vi "AutoLoadRoutines.vi"(1 "Reload Routines":bool, 2 "Auto Routines Storage Directory":path=path "/home/lvuser/AutoRoutines") -> (0 "Auto Routines":T1)   [LabVIEW 2017]
uses:
  TypeDef/AutoRoutines.ctl
  TypeDef/AutoRoutineSet.ctl
  TypeDef/AutoStep.ctl
  TypeDef/AutoWaypointType.ctl
  Pathfinder/Pathfinder-LabVIEW/Pathfinder-Lib/VIs/Waypoint.ctl
  Implements/Arm/TypeDefs/ArmTargetPosition.ctl
  Implements/TypeDefs/IntakeState.ctl
  TypeDef/AutoStartingPositions.ctl
  e61514f7-18c3-42f3-b2a8-fda8a5312ef7.vi
  55916f22-7f41-4e59-abc4-9fcd15d20e92.vi
  058e71e0-aaa7-4a66-86c1-b77b5f723853.vi
  <vilib>/Utility/file.llb/Read Delimited Spreadsheet (DBL).vi
  Pathfinder/Pathfinder-LabVIEW/Pathfinder-Lib/Pathfinder.lvlib
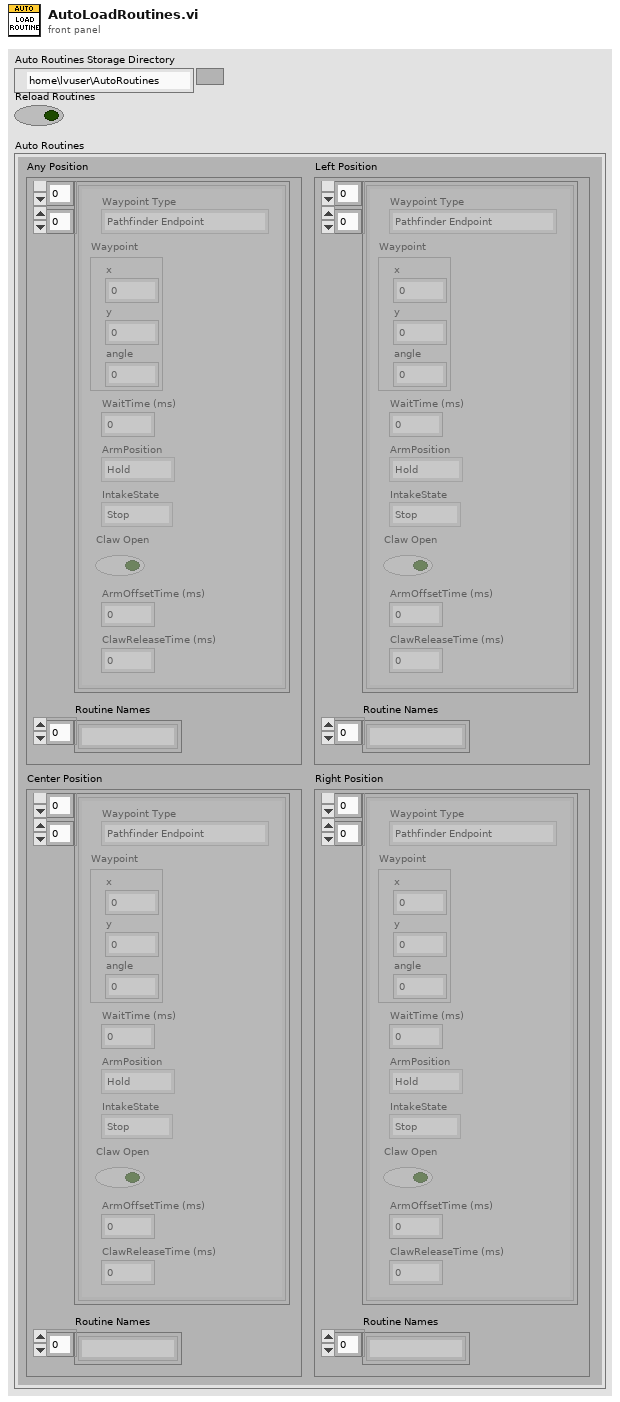
[diagram p1: front panel]
types:
  T1 = typedef "AutoRoutines.ctl" = cluster{"Any Position":T2, "Left Position":T2, "Center Position":T2, "Right Position":T2}
  T2 = typedef "AutoRoutineSet.ctl" = cluster{"Routines":T3[][], "Routine Names":string[]}
  T3 = typedef "AutoStep.ctl" = cluster{"Waypoint Type":T4, "Waypoint":T5, "WaitTime (ms)":u16, "ArmPosition":T6, "IntakeState":T7, "Claw Open":bool, "ArmOffsetTime (ms)":u16, "ClawReleaseTime (ms)":u16}
  T4 = typedef "AutoWaypointType.ctl" = enum16{"Pathfinder Endpoint", "Pathfinder Waypoint", "Zero-Radius Turn Endpoint", "Stationary", "Vision Assist Endpoint", "Stop"}
  T5 = typedef "Pathfinder.lvlib/Waypoint.ctl" = cluster{"x":dbl, "y":dbl, "angle":dbl}
  T6 = typedef "ArmTargetPosition.ctl" = enum16{"Hold", "Switch", "Scale Low", "Scale High", "Climb", "Back Place"}
  T7 = typedef "IntakeState.ctl" = enum16{"Stop", "Forward", "Reverse", "Forward Open"}
  T8 = typedef "AutoStartingPositions.ctl" = enum16{"Any", "Left", "Center", "Right"}
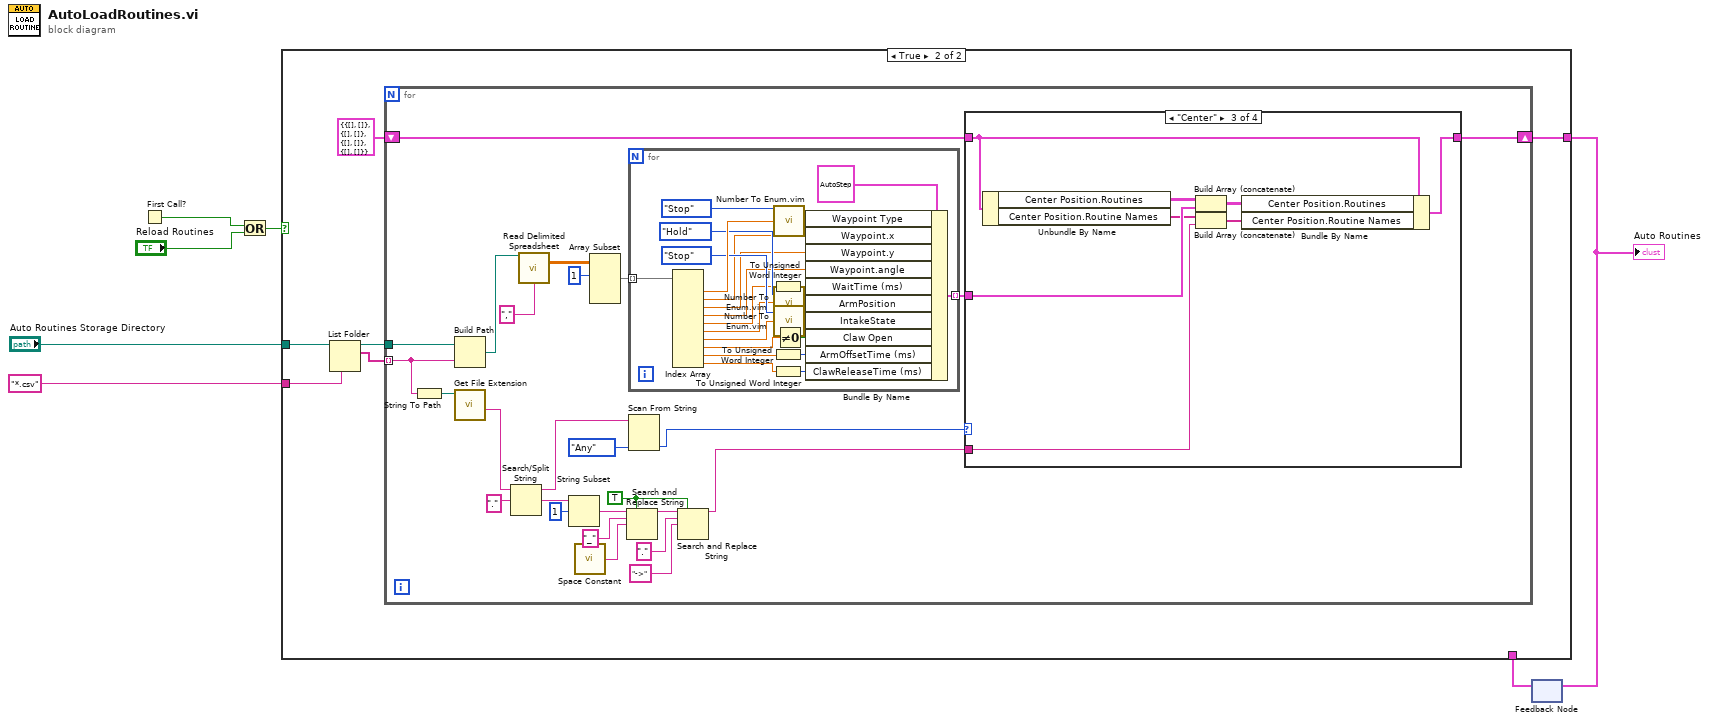
[diagram p0: block diagram]
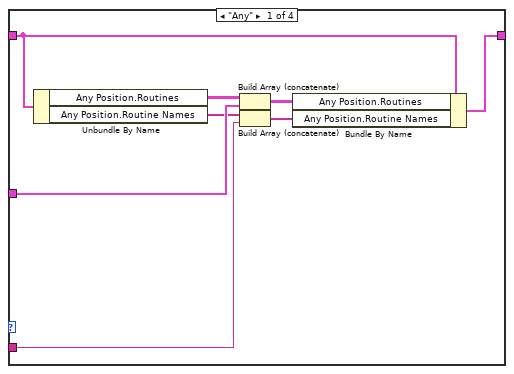
[diagram p3: hidden frame]
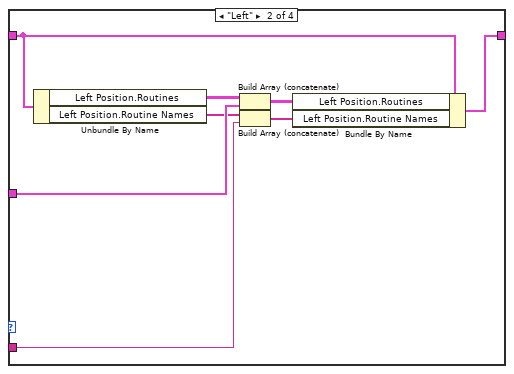
[diagram p4: hidden frame]
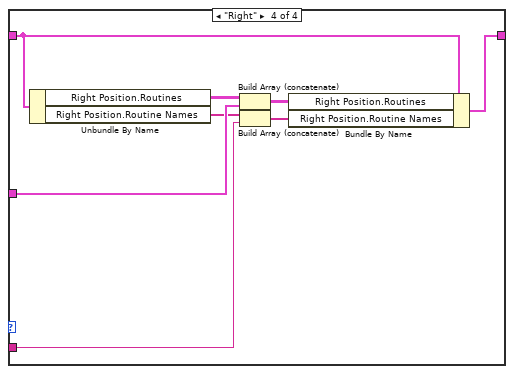
[diagram p5: hidden frame]
diagram:
  n1 = First Call?() -> (First Call?: T/F=w3:bool)
  n2 = Or(x=w3, y="Reload Routines") -> (x .or. y?=w5:bool)
  n3 = feedback #1() -> (w2:T1)  [unwired: 1 in]
  n4 = case shown="True" w5 {
    tunnel: "Auto Routines Storage Directory" -> [_ w14]
    tunnel: "*.csv" ("pattern") -> [_ w13]
    tunnel: [w8 w9] -> w1
    tunnel: w2 -> [w8 _]
    frame False {
    }
    frame True {
      n5 = List Folder(path=w14, pattern=w13) -> (path out=w12:path, filenames=w11:string[])  [unwired: 2 in, 2 out]
      n6 = for {
        tunnel: w12 -> [w37]
        tunnel: w11 -> [w15] mode=indexing
        shift-right: [w17] -> w9
        shift-left: T1 {"Any Position"={"Routines"=[], "Routine Names"=[]}, "Left Position"={"Routines"=[], "Routine Names"=[]}, "Center Position"={"Routines"=[], "Routine Names"=[]}, "Right Position"={"Routines"=[], "Routine Names"=[]}} ("Auto Routine") -> [w19]
        w27 = TRUE ("replace all? (F)")
        n7 = String To Path(string=w15) -> (path=w16:path)
        n8 = Build Path(base path=w37, name or relative path=w15) -> (appended path=w39:path)
        n9 = call <vilib>:"Get File Extension.vi"("file"=w16) -> ("filename without extension"=w36:string)  [unwired: 6 in, 4 out]
        n10 = Search/Split String(string=w36, search string/char (-)=".") -> (substring before match=w22:string, match + rest of string=w35:string)  [unwired: 1 in, 1 out]
        n11 = call-poly <vilib>:"Read Delimited Spreadsheet.vi"("file path (dialog if empty)"=w39, "delimiter (\\t)"="," ("delimiter (\\t)")) -> ("all rows"=w26:dbl[][])  [unwired: 8 in, 5 out]
        n12 = String Subset(string=w35, offset (0)=1) -> (substring=w33:string)  [unwired: 1 in]
        n13 = call <vilib>:"Space Constant.vi"() -> ("String"=w31:string)
        n14 = Array Subset(array=w26, index (row)=1 ("index")) -> (w24:dbl[][])  [unwired: 3 in]
        n15 = Search and Replace String(replace all?=w27, input string=w33, search string="_", replace string=w31) -> (result string=w30:string)  [unwired: 4 in, 3 out]
        n16 = for {
          tunnel: w24 -> [w95] mode=indexing
          tunnel: [w77] -> w18 mode=indexing
          n17 = Index Array(array=w95) -> (element #1=w90:dbl, element #2=w80:dbl, element #3=w79:dbl, element #4=w78:dbl, element #5=w82:dbl, element #6=w84:dbl, element #7=w85:dbl, element #8=w89:dbl, element #9=w76:dbl, element #10=w73:dbl)  [unwired: 10 in]
          n18 = To Unsigned Word Integer(number=w82) -> (unsigned 16bit integer=w81:u16)
          n19 = To Unsigned Word Integer(number=w76) -> (unsigned 16bit integer=w75:u16)
          n20 = To Unsigned Word Integer(number=w73) -> (unsigned 16bit integer=w74:u16)
          n21 = call "Number To Enum.vim"("number"=w90, "enum type"=AutoWaypointType."Stop" ("Waypoint Type")) -> ("number as enum"=w92:T4)
          n22 = call "Number To Enum.vim"("number"=w84, "enum type"=ArmTargetPosition."Hold" ("ArmPosition")) -> ("number as enum"=w86:T6)
          n23 = call "Number To Enum.vim"("number"=w85, "enum type"=IntakeState."Stop" ("IntakeState")) -> ("number as enum"=w88:T7)
          n24 = Not Equal To 0?(x=w89) -> (x != 0?=w93:bool)
          n25 = Bundle By Name(cluster=T3 {"Waypoint Type"=enum."Pathfinder Endpoint", "Waypoint"={"x"=0.0, "y"=0.0, "angle"=0.0}, "WaitTime (ms)"=0, "ArmPosition"=enum."Hold", "IntakeState"=enum."Stop", "Claw Open"=FALSE, "ArmOffsetTime (ms)"=0, "ClawReleaseTime (ms)"=0} ("Cluster"), "Waypoint Type"=w92, "Waypoint.x"=w80, "Waypoint.y"=w79, "Waypoint.angle"=w78, "WaitTime (ms)"=w81, "ArmPosition"=w86, "IntakeState"=w88, "Claw Open"=w93, "ArmOffsetTime (ms)"=w75, "ClawReleaseTime (ms)"=w74) -> (w77:T3)
        }
        n26 = Scan From String(input string=w22, default 1=AutoStartingPositions."Any" ("AutoStartingPosition")) -> (output 1=w20:T8)  [unwired: 3 in, 3 out]
        n27 = Search and Replace String(replace all?=w27, input string=w30, search string=".", replace string="->" ("replace string (\"\")")) -> (result string=w23:string)  [unwired: 4 in, 3 out]
        n28 = case shown="\"Center\"" w20 {
          tunnel: w23 -> [w44 w52 w60 w68]
          tunnel: w19 -> [w48 w56 w64 w72]
          tunnel: w18 -> [w46 w54 w62 w70]
          tunnel: [w41 w49 w57 w65] -> w17
          frame "Any" {
            n29 = Unbundle By Name(w48) -> ("Any Position.Routines"=w47:T3[][], "Any Position.Routine Names"=w45:string[])
            n30 = Build Array (concatenate)(w47, w46) -> (w42:T3[][])
            n31 = Build Array (concatenate)(w45, w44) -> (w43:string[])
            n32 = Bundle By Name(cluster=w48, "Any Position.Routines"=w42, "Any Position.Routine Names"=w43) -> (w41:T1)
          }
          frame "Left" {
            n33 = Unbundle By Name(w56) -> ("Left Position.Routines"=w55:T3[][], "Left Position.Routine Names"=w53:string[])
            n34 = Build Array (concatenate)(w55, w54) -> (w50:T3[][])
            n35 = Build Array (concatenate)(w53, w52) -> (w51:string[])
            n36 = Bundle By Name(cluster=w56, "Left Position.Routines"=w50, "Left Position.Routine Names"=w51) -> (w49:T1)
          }
          frame "Center" {
            n37 = Unbundle By Name(w64) -> ("Center Position.Routines"=w63:T3[][], "Center Position.Routine Names"=w61:string[])
            n38 = Build Array (concatenate)(w63, w62) -> (w58:T3[][])
            n39 = Build Array (concatenate)(w61, w60) -> (w59:string[])
            n40 = Bundle By Name(cluster=w64, "Center Position.Routines"=w58, "Center Position.Routine Names"=w59) -> (w57:T1)
          }
          frame "Right" {
            n41 = Unbundle By Name(w72) -> ("Right Position.Routines"=w71:T3[][], "Right Position.Routine Names"=w69:string[])
            n42 = Build Array (concatenate)(w71, w70) -> (w66:T3[][])
            n43 = Build Array (concatenate)(w69, w68) -> (w67:string[])
            n44 = Bundle By Name(cluster=w72, "Right Position.Routines"=w66, "Right Position.Routine Names"=w67) -> (w65:T1)
          }
        }
      }
    }
  }
  "Auto Routines" <- w1
  n45 = feedback-in #1(w1) -> ()
